vi "scil_reg2.vi"() -> ()   [LabVIEW 2010]
uses:
  glob1.vi
  <instrlib>/niSync/niSync.llb/niSync Initialize (String).vi
panel:
  in  "Path":path
  in  "test":bool=TRUE
  out "ahtung":bool
  out "seconds_remind":dbl(knob) scale=0.0..110.0
  in  "stop":bool
  out "found":bool
  out "nearest":timestamp
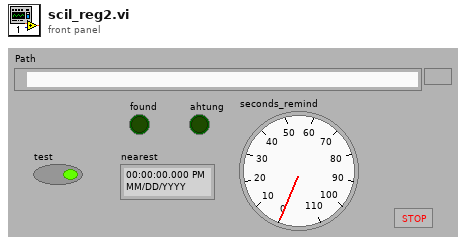
[diagram p1: front panel]
types:
  T1 = typedef "niScope vertical coupling.ctl" = i32
  T2 = cluster{"channel name":string, "input impedance":u32, "maximum input frequency":dbl, "vertical coupling":T1, "probe attenuation":dbl, "vertical range":dbl, "vertical offset":dbl, "channel enabled":bool}[]
  T3 = cluster{"channel name":string, "input impedance":u32, "maximum input frequency":dbl, "vertical coupling":T1, "probe attenuation":dbl, "vertical range":dbl, "vertical offset":dbl, "channel enabled":bool}
  T4 = cluster{"enforce realtime":bool, "number of records":i32, "min sample rate":dbl, "reference position":dbl, "min record length":i32}
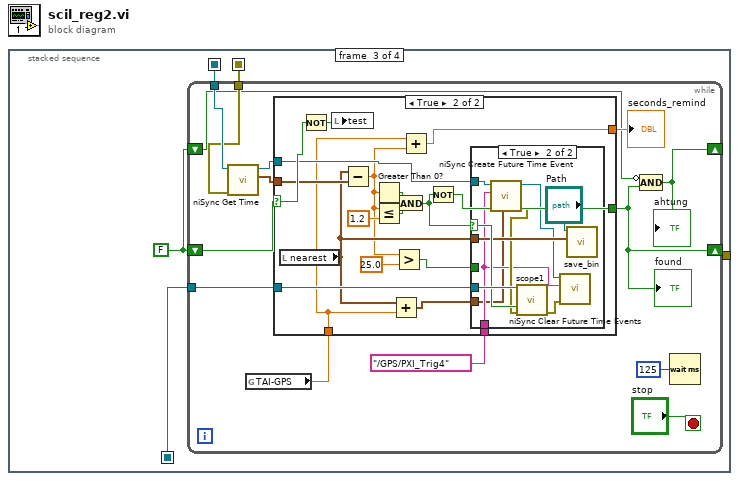
[diagram p0: block diagram]
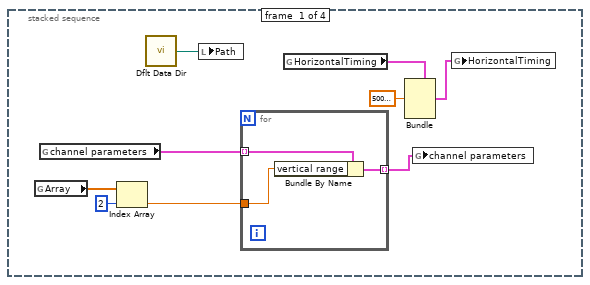
[diagram p2: hidden frame]
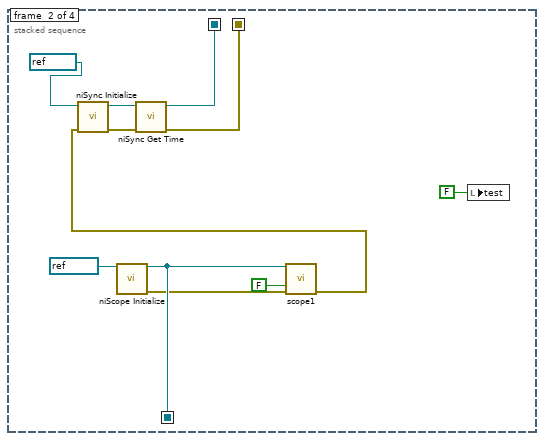
[diagram p3: hidden frame]
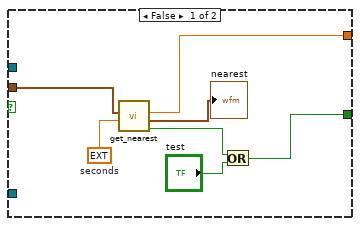
[diagram p4: hidden frame]
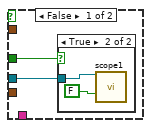
[diagram p5: hidden frame]
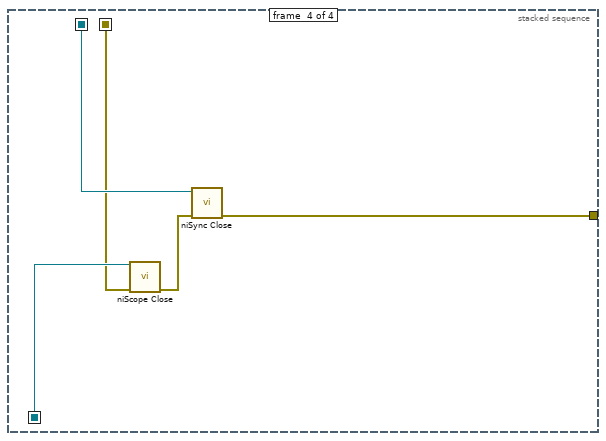
[diagram p7: hidden frame]
diagram:
  n1 = stacked-sequence {
    seq-local: [_ w20 _ _] -> [_ _ w25 w85]
    seq-local: [_ w19 _ _] -> [_ _ w24 w82]
    seq-local: [_ w17 _ _] -> [_ _ w26 w83]
    tunnel: [_ _ _ w84] -> _
    frame #0 {
      n2 = global read "glob1.vi" "Array"() -> (w7:dbl[])
      n3 = global read "glob1.vi" "channel parameters"() -> (w9:T2)
      n4 = Index Array(array=w7, index=2) -> (element=w5:dbl)
      n5 = call <vilib>:"Dflt Data Dir.vi"() -> ("App:Default Data Directory"=w4:path)
      n6 = local write "Path"(w4) -> ()
      n7 = for {
        tunnel: w9 -> [w12] mode=indexing
        tunnel: [w11] -> w8 mode=indexing
        tunnel: w5 -> [w10]
        n8 = Bundle By Name(cluster=w12, "vertical range"=w10) -> (w11:T3)
      }
      n9 = global read "glob1.vi" "HorizontalTiming"() -> (w3:T4)
      n10 = Bundle(cluster=w3, "min sample rate"=50000000.0) -> (w2:T4)  [unwired: 4 in]
      n11 = global write "glob1.vi" "channel parameters"(w8) -> ()
      n12 = global write "glob1.vi" "HorizontalTiming"(w2) -> ()
    }
    frame #1 {
      n13 = call <instrlib>:"niScope Initialize.vi"("resource name"=refnum<k15> "ADC") -> ("instrument handle"=w17:refnum<k15>, "error out"=w16:errorcluster)  [unwired: 13 in]
      n14 = call "scope1.vi"("instrument handle"=w17, "TriggerMode"=FALSE, "error in"=w16) -> ("error out"=w14:errorcluster)  [unwired: 11 in, 1 out]
      n15 = call-poly <instrlib>:"niSync Initialize.vi"("error in (no error)"=w14, "resource name"=refnum<k15> "GPS" ("IVI Logical Name")) -> ("error out"=w22:errorcluster, "instrument handle out"=w21:refnum<k15>)  [unwired: 8 in]
      n16 = call <instrlib>:"niSync Get Time.vi"("error in (no error)"=w22, "instrument handle"=w21) -> ("error out"=w19:errorcluster, "instrument handle out"=w20:refnum<k15>)  [unwired: 5 in, 1 out]
      n17 = local write "test"(FALSE ("test")) -> ()
    }
    frame #2 {
      w27 = FALSE ("found")
      n18 = while {
        shift-right: [w31] -> _
        shift-left: w27 -> [w38]
        shift-right: [w30] -> _
        shift-left: w27 -> [w29]
        tunnel: w26 -> [w37]
        tunnel: w25 -> [w35]
        tunnel: w24 -> [w32]
        stop <- "stop" stop-if-true
        n19 = call <instrlib>:"niSync Get Time.vi"("error in (no error)"=w32, "instrument handle"=w35) -> ("time"=w33:timestamp, "instrument handle out"=w34:refnum<k15>)  [unwired: 5 in, 1 out]
        n20 = global read "glob1.vi" "TAI-GPS"() -> (w28:dbl)
        n21 = case shown="True" w38 {
          selector: w38 -> [_ w58]
          tunnel: [w43 w65] -> w31
          tunnel: [w46 w50] -> w39
          tunnel: w37 -> [_ w57]
          tunnel: tag "/GPS/PXI_Trig4" ("terminal") -> [_ w56]
          tunnel: w34 -> [_ w55]
          tunnel: w33 -> [w42 w54]
          tunnel: w28 -> [_ w49]
          frame False {
            w47 = ext 120.0  # seconds
            n22 = call "get_nearest.vi"("interval_sec"=w47, "current time"=w42) -> ("found"=w45:bool, "next_TimeStamp"=→"nearest":timestamp, "seconds_remind"=w46:dbl)  [unwired: 3 in]
            n23 = Or(x=w45, y="test") -> (x .or. y?=w43:bool)
          }
          frame True {
            n24 = local read "nearest"() -> (w53:timestamp)
            n25 = Not(x=w58) -> (.not. x?=w59:bool)
            n26 = local write "test"(w59) -> ()
            n27 = Subtract(x=w53, y=w54) -> (x-y=w51:dbl)
            n28 = Greater Than 0?(x=w51) -> (x > 0?=w63:bool)
            n29 = Less Or Equal?(x=w51, y=1.2) -> (x <= y?=w64:bool)
            n30 = Add(x=w53, y=w49) -> (x+y=w52:timestamp)
            n31 = Greater?(x=w51, y=25.0) -> (0:w60:bool)
            n32 = And(x=w63, y=w64) -> (x .and. y?=w62:bool)
            n33 = Add(x=w49, y=w51) -> (x+y=w50:dbl)
            n34 = Not(x=w62) -> (.not. x?=w65:bool)
            n35 = case shown="True" w62 {
              selector: w62 -> [_ w78]
              tunnel: w53 -> [_ w77]
              tunnel: w60 -> [w68 _]
              tunnel: w57 -> [w67 w80]
              tunnel: w55 -> [_ w75]
              tunnel: w56 -> [_ w72]
              tunnel: w52 -> [_ w71]
              frame False {
                n36 = case shown="True" w68 {
                  tunnel: w67 -> [_ w70]
                  frame False {
                  }
                  frame True {
                    n37 = call "scope1.vi"("instrument handle"=w70, "TriggerMode"=FALSE) -> ()  [unwired: 12 in, 2 out]
                  }
                }
              }
              frame True {
                n38 = call <instrlib>:"niSync Create Future Time Event.vi"("time"=w71, "terminal"=w72, "instrument handle"=w75) -> ("error out"=w76:errorcluster, "instrument handle out"=w73:refnum<k15>)  [unwired: 6 in]
                n39 = call "scope1.vi"("instrument handle"=w80, "TriggerMode"=w78, "error in"=w76) -> ("error out"=w74:errorcluster)  [unwired: 11 in, 1 out]
                n40 = call <instrlib>:"niSync Clear Future Time Events.vi"("error in (no error)"=w74, "terminal"=w72, "instrument handle"=w73) -> ()  [unwired: 6 in, 2 out]
                n41 = call "save_bin.vi"("timestamp"=w77, "start path"="Path") -> ()  [unwired: 4 in, 2 out]
              }
            }
          }
        }
        "found" <- w31
        "seconds_remind" <- w39
        n42 = Compound Arithmetic op=AND(invert w29, w31) -> (w30:bool)
        "ahtung" <- w30
        n43 = Wait (ms)(milliseconds to wait=u32 125) -> ()  [unwired: 1 out]
      }
    }
    frame #3 {
      n44 = call <instrlib>:"niScope Close.vi"("instrument handle"=w83, "error in"=w82) -> ("error out"=w81:errorcluster)  [unwired: 13 in]
      n45 = call <instrlib>:"niSync Close.vi"("error in (no error)"=w81, "instrument handle"=w85) -> ("error out"=w84:errorcluster)  [unwired: 9 in]
    }
  }
